vi "Run.vi"(8 "error in (no error)":errorcluster, 10 "Buffer Size":u64=2048, 11 "Mixer in":refnum<class "Mixer.lvclass">) -> (0 "error out":errorcluster, 3 "Mixer out":refnum<class "Mixer.lvclass">)   [LabVIEW 2020, in "G-Audio.lvlib" / "Mixer.lvclass"]
uses:
  Mixer.lvclass
  Mixer.lvclass/Mixer.ctl
  6b6e21db-26d8-44fc-bcc7-090b1c1e96ee.vi
  Private/Result To Error.vi
  6b6e21db-26d8-44fc-bcc7-090b1c1e96ee.vi/4dfb5711-8d81-45a3-b3db-a84d40650863.vi
  6b6e21db-26d8-44fc-bcc7-090b1c1e96ee.vi/c8869513-30c6-44f2-a2d3-73232fe63870.vi
  6b6e21db-26d8-44fc-bcc7-090b1c1e96ee.vi/4dfb5711-8d81-45a3-b3db-a84d40650863.vi/53d6f456-6d93-41d3-8485-27023fbbbc96.vi
  6b6e21db-26d8-44fc-bcc7-090b1c1e96ee.vi/c8869513-30c6-44f2-a2d3-73232fe63870.vi/53d6f456-6d93-41d3-8485-27023fbbbc96.vi
  <vilib>/Utility/Data Type/Get Numeric Information.vi
  <vilib>/Utility/error.llb/Error Cluster From Error Code.vi
  Channel/Channel.lvclass
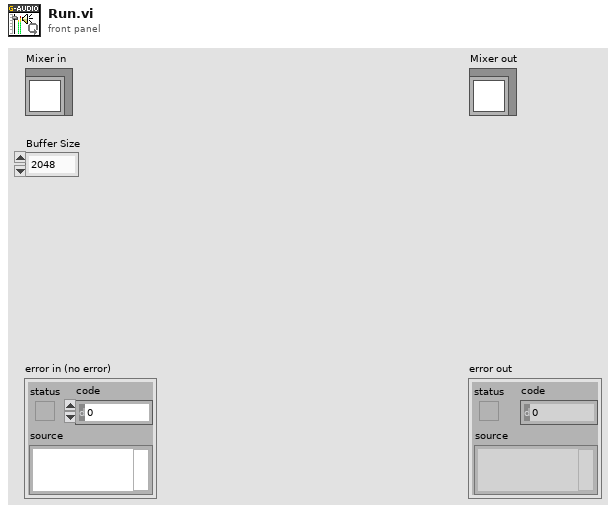
[diagram p1: front panel]
types:
  T1 = typedef "G-Audio.lvlib/Audio Device Refnum.ctl" = refnum<file>
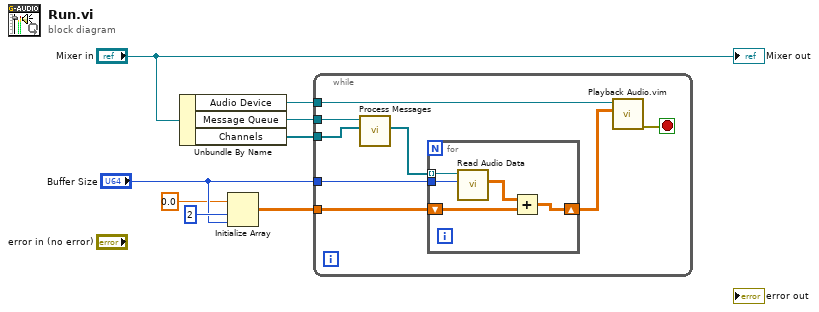
[diagram p0: block diagram]
diagram:
  n1 = Unbundle By Name("Mixer in") -> ("Audio Device"=w8:T1, "Message Queue"=w1:refnum<queue>, "Channels"=w7:refnum<data-value>[])
  n2 = Initialize Array(sgl 0.0 ("element"), u64 2 ("dimension size"), "Buffer Size") -> (w5:sgl[][])
  n3 = while {
    tunnel: w8 -> [w16]
    tunnel: w7 -> [w10]
    tunnel: w5 -> [w15]
    tunnel: "Buffer Size" -> [w12]
    tunnel: w1 -> [w11]
    stop <- w13 stop-if-true
    n4 = call "Process Messages.vi"("Channels in"=w10, "Message Queue"=w11) -> ("Channels out"=w9:refnum<data-value>[])  [unwired: 9 in]
    n5 = for {
      tunnel: w9 -> [w17] mode=indexing
      shift-right: [w21] -> w14
      shift-left: w15 -> [w20]
      tunnel: w12 -> [w18]
      n6 = call "Read Audio Data.vi"("Frames"=w18, "Channel in"=w17) -> ("Audio Data"=w19:sgl[][])  [unwired: 7 in, 2 out]
      n7 = Add(x=w19, y=w20) -> (x+y=w21:sgl[][])
    }
    n8 = call "Playback Audio.vim"("Audio Data"=w14, "Audio Device Refnum In"=w16) -> ("error out"=w13:errorcluster)  [unwired: 8 in, 1 out]
  }
  "Mixer out" <- "Mixer in"
